vi "Snapshot Viewer.vi"() -> ()   [LabVIEW 2017]
uses:
  MainArray.ctl
panel:
  out "data":T1
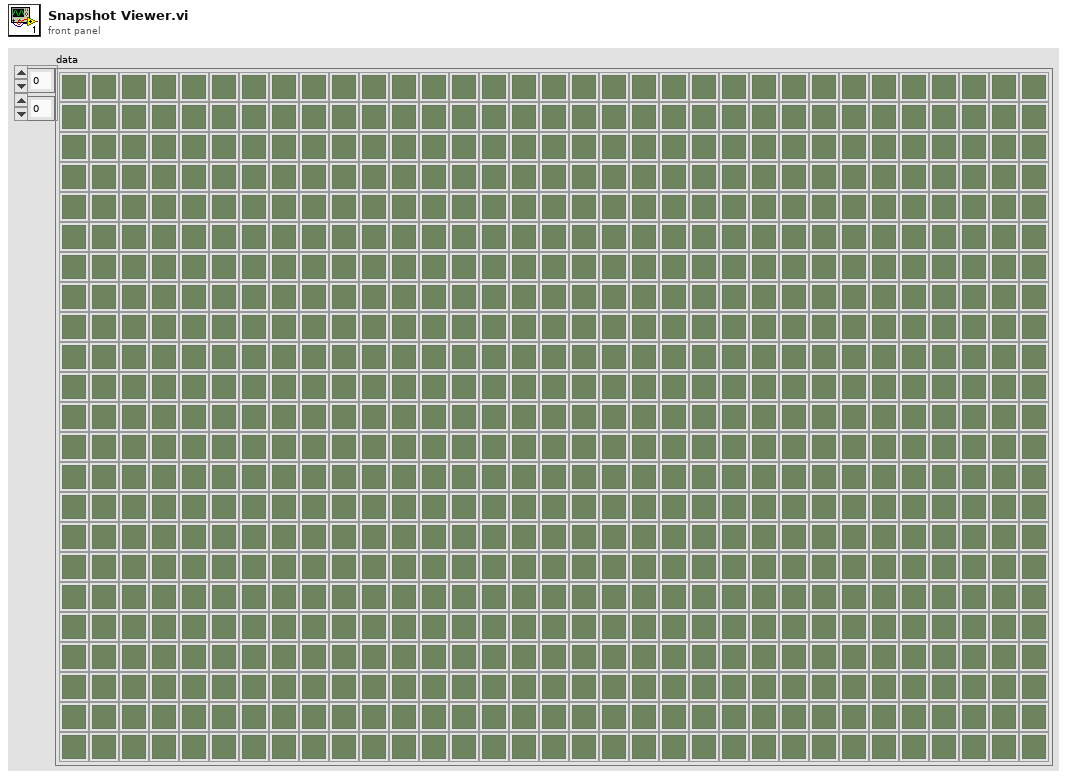
[diagram p1: front panel]
types:
  T1 = typedef "MainArray.ctl" = bool[][]
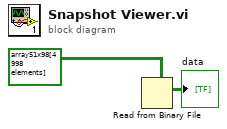
[diagram p0: block diagram]
diagram:
  n1 = Read from Binary File(5:T1 array51x98[4998 elements] ("Array")) -> (2:→"data":T1)  [unwired: 5 in, 3 out]
